vi "copy.vi"(8 "error in (no error)":errorcluster, 10 "ScriptEventForCopy":refnum<class "ScriptEvent.lvclass">, 11 "SingleTone in":refnum<class "SingleTone.lvclass">) -> (0 "error out":errorcluster, 3 "SingleTone Copy":refnum<class "SingleTone.lvclass">)   [LabVIEW 2011, in "Tools.lvlib" / "Scripting.lvlib" / "SingleTone.lvclass"]
uses:
  SingleTone.lvclass
  ScriptEvent.lvclass
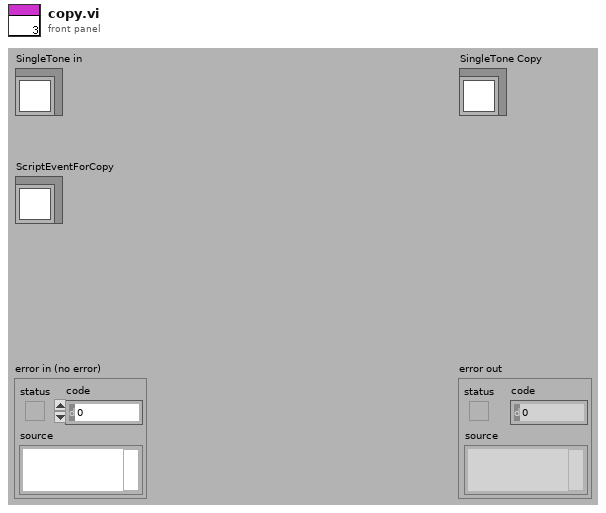
[diagram p1: front panel]
types:
  T1 = enum16{"changeValue", "pulse", "clock", "rampUp", "rampDown", "singleTone", "singleToneRamp", "playFile", "rf", "rfRamp", "delay"}
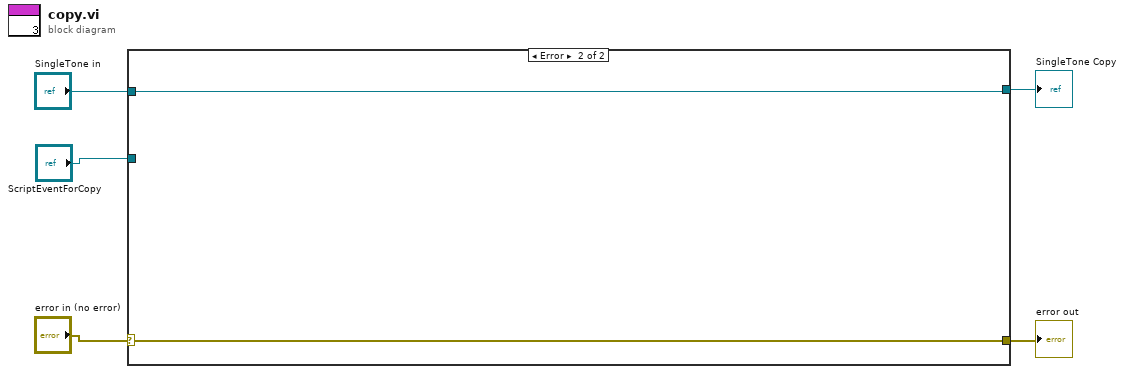
[diagram p0: block diagram]
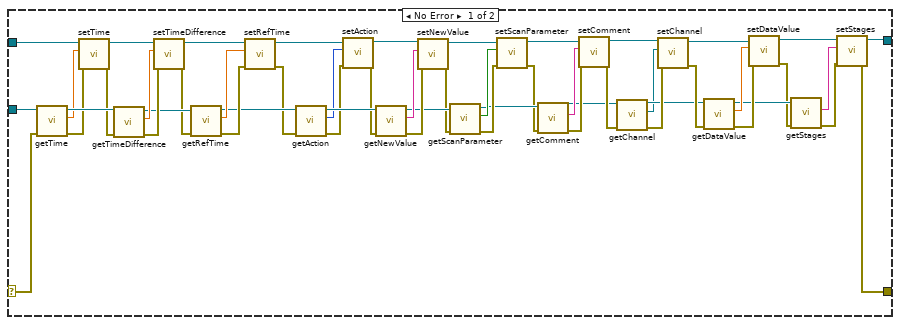
[diagram p2: hidden frame]
diagram:
  n1 = case shown="Error" "error in (no error)" {
    selector: "error in (no error)" -> [w19 w59]
    tunnel: [w7 w58] -> w5
    tunnel: [w6 w59] -> w4
    tunnel: "SingleTone in" -> [w9 w58]
    tunnel: "ScriptEventForCopy" -> [w8 _]
    frame No Error {
      n2 = call "getTime.vi"("error in (no error)"=w19, "ScriptEvent.lvclass in"=w8) -> ("error out"=w56:errorcluster, "time"=w55:dbl, "ScriptEvent.lvclass out"=w57:refnum<class "ScriptEvent.lvclass">)  [unwired: 7 in]
      n3 = call "setTime.vi"("error in (no error)"=w56, "time"=w55, "ScriptEvent.lvclass in"=w9) -> ("error out"=w54:errorcluster, "ScriptEvent.lvclass out"=w26:refnum<class "SingleTone.lvclass">)  [unwired: 7 in]
      n4 = call "getTimeDifference.vi"("error in (no error)"=w54, "ScriptEvent.lvclass in"=w57) -> ("error out"=w53:errorcluster, "time difference"=w27:dbl, "ScriptEvent.lvclass out"=w15:refnum<class "ScriptEvent.lvclass">)  [unwired: 7 in]
      n5 = call "setTimeDifference.vi"("error in (no error)"=w53, "time difference"=w27, "ScriptEvent.lvclass in"=w26) -> ("error out"=w14:errorcluster, "ScriptEvent.lvclass out"=w16:refnum<class "SingleTone.lvclass">)  [unwired: 7 in]
      n6 = call "getRefTime.vi"("error in (no error)"=w14, "ScriptEvent.lvclass in"=w15) -> ("error out"=w12:errorcluster, "refTime"=w13:dbl, "ScriptEvent.lvclass out"=w11:refnum<class "ScriptEvent.lvclass">)  [unwired: 7 in]
      n7 = call "setRefTime.vi"("error in (no error)"=w12, "refTime"=w13, "ScriptEvent.lvclass in"=w16) -> ("error out"=w10:errorcluster, "ScriptEvent.lvclass out"=w17:refnum<class "SingleTone.lvclass">)  [unwired: 7 in]
      n8 = call "getAction.vi"("error in (no error)"=w10, "ScriptEvent.lvclass in"=w11) -> ("error out"=w51:errorcluster, "action"=w50:T1, "ScriptEvent.lvclass out"=w52:refnum<class "ScriptEvent.lvclass">)  [unwired: 7 in]
      n9 = call "setAction.vi"("error in (no error)"=w51, "action"=w50, "ScriptEvent.lvclass in"=w17) -> ("error out"=w49:errorcluster, "ScriptEvent.lvclass out"=w25:refnum<class "SingleTone.lvclass">)  [unwired: 7 in]
      n10 = call "getNewValue.vi"("error in (no error)"=w49, "ScriptEvent.lvclass in"=w52) -> ("error out"=w48:errorcluster, "newValue"=w47:string, "ScriptEvent.lvclass out"=w46:refnum<class "ScriptEvent.lvclass">)  [unwired: 7 in]
      n11 = call "setNewValue.vi"("error in (no error)"=w48, "newValue"=w47, "ScriptEvent.lvclass in"=w25) -> ("error out"=w45:errorcluster, "ScriptEvent.lvclass out"=w24:refnum<class "SingleTone.lvclass">)  [unwired: 7 in]
      n12 = call "getScanParameter.vi"("error in (no error)"=w45, "ScriptEvent.lvclass in"=w46) -> ("error out"=w43:errorcluster, "scanParameter"=w44:bool, "ScriptEvent.lvclass out"=w42:refnum<class "ScriptEvent.lvclass">)  [unwired: 7 in]
      n13 = call "setScanParameter.vi"("error in (no error)"=w43, "scanParameter"=w44, "ScriptEvent.lvclass in"=w24) -> ("error out"=w41:errorcluster, "ScriptEvent.lvclass out"=w23:refnum<class "SingleTone.lvclass">)  [unwired: 7 in]
      n14 = call "getComment.vi"("error in (no error)"=w41, "ScriptEvent.lvclass in"=w42) -> ("error out"=w40:errorcluster, "comment"=w39:string, "ScriptEvent.lvclass out"=w37:refnum<class "ScriptEvent.lvclass">)  [unwired: 7 in]
      n15 = call-dynamic "setComment.vi"("error in (no error)"=w40, "comment"=w39, "ScriptEvent.lvclass in"=w23) -> ("error out"=w38:errorcluster, "ScriptEvent.lvclass out"=w22:refnum<class "SingleTone.lvclass">)  [unwired: 7 in]
      n16 = call-dynamic "getChannel.vi"("error in (no error)"=w38, "ScriptEvent.lvclass in"=w37) -> ("error out"=w36:errorcluster, "Channel.lvclass"=w18:refnum<class "Channel.lvclass">, "ScriptEvent.lvclass out"=w34:refnum<class "ScriptEvent.lvclass">)  [unwired: 7 in]
      n17 = call-dynamic "setChannel.vi"("error in (no error)"=w36, "Channel.lvclass"=w18, "ScriptEvent.lvclass in"=w22) -> ("error out"=w35:errorcluster, "ScriptEvent.lvclass out"=w21:refnum<class "SingleTone.lvclass">)  [unwired: 7 in]
      n18 = call "getDataValue.vi"("error in (no error)"=w35, "ScriptEvent.lvclass in"=w34) -> ("error out"=w33:errorcluster, "dataValue"=w32:dbl, "ScriptEvent.lvclass out"=w31:refnum<class "ScriptEvent.lvclass">)  [unwired: 7 in]
      n19 = call "setDataValue.vi"("error in (no error)"=w33, "dataValue"=w32, "ScriptEvent.lvclass in"=w21) -> ("error out"=w30:errorcluster, "ScriptEvent.lvclass out"=w20:refnum<class "SingleTone.lvclass">)  [unwired: 7 in]
      n20 = call "getStages.vi"("error in (no error)"=w30, "ScriptEvent.lvclass in"=w31) -> ("error out"=w29:errorcluster, "Stage"=w28:string)  [unwired: 7 in, 1 out]
      n21 = call-dynamic "setStages.vi"("error in (no error)"=w29, "Stage"=w28, "ScriptEvent.lvclass in"=w20) -> ("error out"=w6:errorcluster, "ScriptEvent.lvclass out"=w7:refnum<class "SingleTone.lvclass">)  [unwired: 7 in]
    }
    frame Error {
    }
  }
  "error out" <- w4
  "SingleTone Copy" <- w5
